vi "Create Failure Data.vi"(7 "System Time":dbl[](array[numeric]), 8 "error in (no error)":errorcluster, 9 "Idx":i32, 10 "Graph Data":dbl[][](array[numeric]), 11 "Test Data":T1[](array[typedef])) -> (0 "error out":errorcluster, 1 "MultiLB Data":string[][](array[string]), 2 "Graph Data dup":dbl[][](array[numeric]))   [LabVIEW 2011]
uses:
  Controls/Test Column Data.ctl
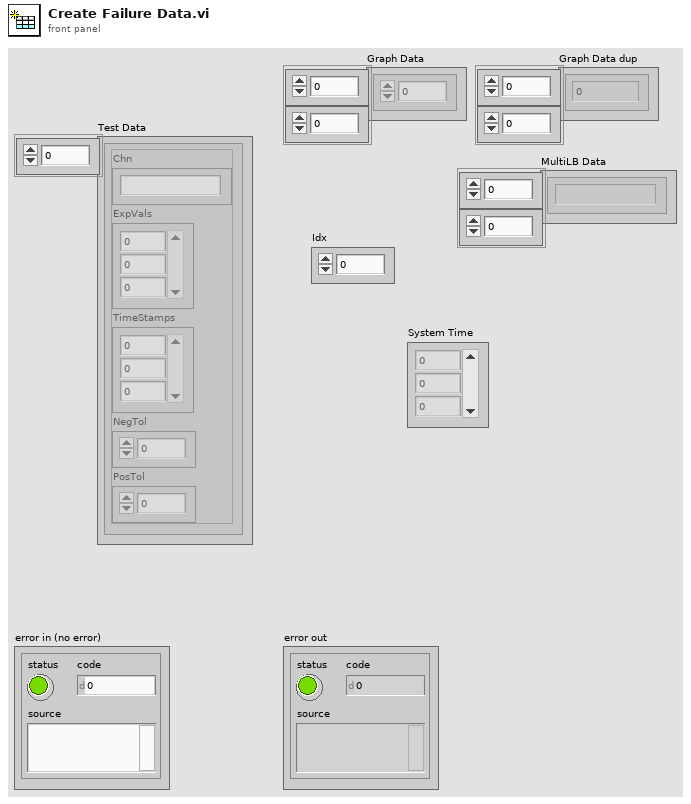
[diagram p1: front panel]
types:
  T1 = typedef "Test Column Data.ctl" = cluster{"Chn":string, "ExpVals":dbl[], "TimeStamps":i64[], "NegTol":dbl, "PosTol":dbl}
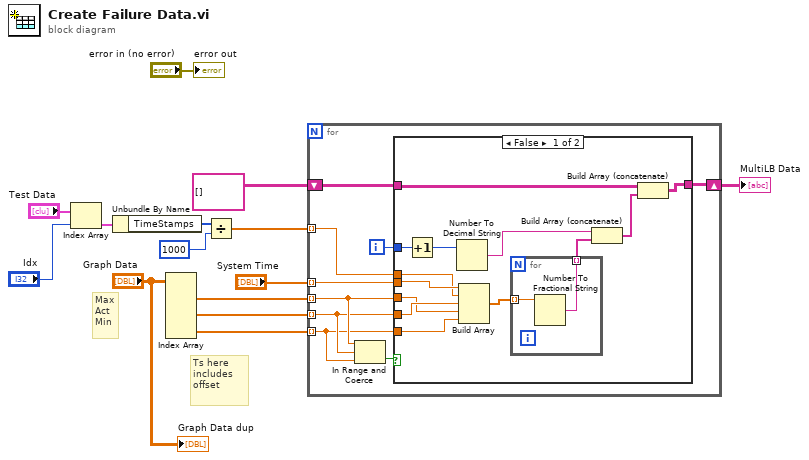
[diagram p0: block diagram]
diagram:
  # "Max\nAct\nMin"
  # "Ts here includes offset"
  n1 = Index Array(array="Test Data", index="Idx") -> (element=w14:T1)
  n2 = Unbundle By Name(w14) -> ("TimeStamps"=w12:i64[])
  n3 = Index Array(array="Graph Data") -> (element #1=w2:dbl[], element #2=w11:dbl[], element #3=w3:dbl[])  [unwired: 6 in]
  n4 = Divide(x=w12, y=i64 1000 ("x")) -> (x/y=w10:dbl[])
  n5 = for {
    tunnel: w10 -> [w16] mode=indexing
    shift-right: [w22] -> w4
    shift-left: string[][] [] -> [w23]
    tunnel: w3 -> [w17] mode=indexing
    tunnel: w11 -> [w18] mode=indexing
    tunnel: w2 -> [w19] mode=indexing
    tunnel: "System Time" -> [w15] mode=indexing
    i -> [w21]
    n6 = In Range and Coerce(upper limit=w19, x=w18, lower limit=w17) -> (In Range?=w20:bool)  [unwired: 1 out]
    n7 = case shown="False" w20 {
      tunnel: w23 -> [w36 w39]
      tunnel: [w35 w39] -> w22
      tunnel: w17 -> [w28 _]
      tunnel: w18 -> [w27 _]
      tunnel: w19 -> [w26 _]
      tunnel: w21 -> [w34 _]
      tunnel: w16 -> [w24 _]
      tunnel: w15 -> [w25 _]
      frame False {
        n8 = Increment(x=w34) -> (x+1=w31:i32)
        n9 = Number To Decimal String(number=w31) -> (decimal integer string=w30:string)  [unwired: 1 in]
        n10 = Build Array(w25, w24, w27, w26, w28) -> (w33:dbl[])
        n11 = for {
          tunnel: w33 -> [w38] mode=indexing
          tunnel: [w37] -> w32 mode=indexing
          n12 = Number To Fractional String(number=w38) -> (F-format string=w37:string)  [unwired: 3 in]
        }
        n13 = Build Array (concatenate)(w30, w32) -> (w29:string[])
        n14 = Build Array (concatenate)(w36, w29) -> (w35:string[][])
      }
      frame True {
      }
    }
  }
  "MultiLB Data" <- w4
  "error out" <- "error in (no error)"
  "Graph Data dup" <- "Graph Data"
